vi "Begin.vi"(8 "error in (no error)":errorcluster, 11 "Dev Grabber in":refnum<class "Dev Grabber.lvclass">) -> (0 "error out":errorcluster, 3 "Dev Grabber out":refnum<class "Dev Grabber.lvclass">)   [LabVIEW 2014, in "Dev Grabber.lvlib" / "Dev Grabber.lvclass"]
uses:
  Dev Grabber.lvclass
  <vilib>/Rock Robotics/WPI/CAN/TalonSRX/WPI_CANTalonSRX_APIControlMode.ctl
  Dev Grabber.lvclass/Dev Grabber.ctl
  <vilib>/Rock Robotics/WPI/Solenoid/WPI_SolenoidOpenDouble.vi
  <vilib>/Rock Robotics/WPI/MotorControl/WPI_MotorControlOpenCANTalonSRX.vi
  Robot/Grabber/Grabber Class/Grabber.lvclass
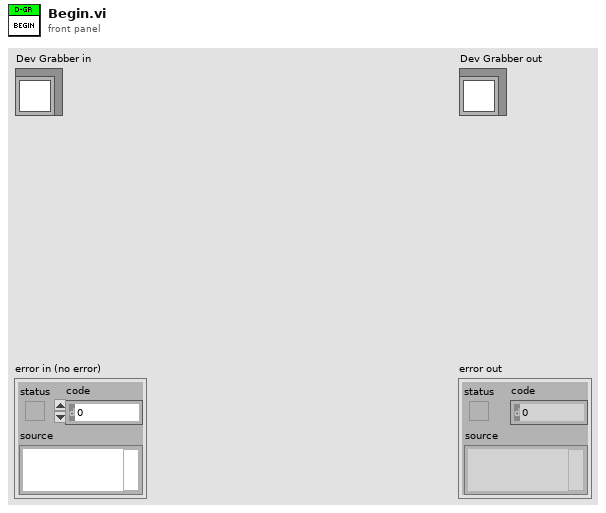
[diagram p1: front panel]
types:
  T1 = typedef "WPI_CANTalonSRX_APIControlMode.ctl" = enum8{"Percent VBus", "Speed", "Position", "Slave", "Unchanged / Invalid"}
  T2 = typedef "WPI_SolenoidChannel.ctl" = enum8{"Solenoid 0", "Solenoid 1", "Solenoid 2", "Solenoid 3", "Solenoid 4", "Solenoid 5", "Solenoid 6", "Solenoid 7", "Invalid"}
  T3 = typedef "WPI_SolenoidDevRef.ctl" = cluster{"DevStatus":errorcluster, "Pneumatics Control Module":u8, "Forward Solenoid Channel":T2, "Reverse Solenoid Channel":T2}
  T4 = typedef "WPI_MotorControlDeviceRef.ctl" = cluster{"DeviceStatus":errorcluster, "Type":T5, "PWM":cluster{"Controller":T6, "PWM Channel":T7, "DeadBand":T8}, "CAN":cluster{"Device Number":u8, "Control Mode":T9, "Semaphore":T10, "Max Vout":dbl, "TalonSRX Control Mode":T1}, "Invert":bool, "TransformRef":T11, "InvTransformRef":T11}
  T5 = typedef "WPI_MotorControlType.ctl" = enum16{"PWM", "CAN", "CANTalonSRX"}
  T6 = typedef "FPGA_TypedefDigitalModule.ctl" = enum16{"Controller 1"}
  T7 = typedef "FPGA_DIOPWMChannel.ctl" = enum8{"PWM 0", "PWM 1", "PWM 2", "PWM 3", "PWM 4", "PWM 5", "PWM 6", "PWM 7", "PWM 8", "PWM 9", "PWM MXP 0", "PWM MXP 1", "PWM MXP 2", "PWM MXP 3", "PWM MXP 4", "PWM MXP 5", "PWM MXP 6", "PWM MXP 7", "PWM MXP 8", "PWM MXP 9", "Invalid"}
  T8 = typedef "WPI_PWMDeadband.ctl" = cluster{"Name":string, "maxPositivePwm":i32, "minPositivePwm":i32, "centerPwm":i32, "maxNegativePwm":i32, "minNegativePwm":i32, "angularRange":u16}
  T9 = typedef "WPI_CANJaguar_ControlMode.ctl" = enum8{"Percent VBus", "Current", "Speed", "Position", "Voltage"}
  T10 = typedef "Semaphore RefNum" = refnum<k1>
  T11 = typedef "WPI_PWMTransform_ConPane.ctl" = refnum<vi>
  T12 = typedef "Dev Grabber.lvlib/Dev Grabber.lvclass/Dev Grabber Config.ctl" = cluster{"PCM CAN ID":u8, "Forward Solenoid Channel":T2, "Reverse Solenoid Channel":T2, "Left Motor CAN ID":u8, "Right Motor CAN ID":u8, "Left Motor Invert":bool, "Right Motor Invert":bool}
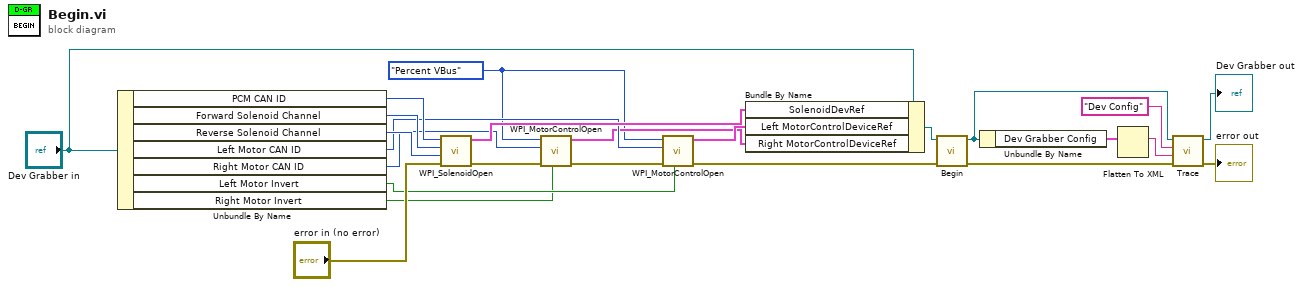
[diagram p0: block diagram]
diagram:
  w11 = WPI_CANTalonSRX_APIControlMode."Percent VBus" ("Control Mode")
  n1 = Unbundle By Name("Dev Grabber in") -> ("PCM CAN ID"=w23:u8, "Forward Solenoid Channel"=w22:T2, "Reverse Solenoid Channel"=w21:T2, "Left Motor CAN ID"=w17:u8, "Right Motor CAN ID"=w14:u8, "Left Motor Invert"=w16:bool, "Right Motor Invert"=w13:bool)
  n2 = call-poly <vilib>:"WPI_SolenoidOpen.vi"("error in (no error)"="error in (no error)", "Reverse Solenoid Channel"=w21, "Forward Solenoid Channel"=w22, "Pneumatics Control Module (0)"=w23) -> ("error out"=w10:errorcluster, "SolenoidDevRef"=w19:T3)  [unwired: 6 in]
  n3 = call-poly <vilib>:"WPI_MotorControlOpen.vi"("Invert"=w13, "error in (no error)"=w10, "Device Number"=w14, "Control Mode"=w11) -> ("error out"=w9:errorcluster, "MotorControlDeviceRef"=w12:T4)  [unwired: 6 in]
  n4 = call-poly <vilib>:"WPI_MotorControlOpen.vi"("Invert"=w16, "error in (no error)"=w9, "Device Number"=w17, "Control Mode"=w11) -> ("error out"=w8:errorcluster, "MotorControlDeviceRef"=w15:T4)  [unwired: 6 in]
  n5 = Bundle By Name(cluster="Dev Grabber in", "SolenoidDevRef"=w19, "Left MotorControlDeviceRef"=w15, "Right MotorControlDeviceRef"=w12) -> (w20:refnum<class "Dev Grabber.lvclass">)
  n6 = call-parent "Begin.vi"("error in (no error)"=w8, "System Actor in"=w20) -> ("error out"=w6:errorcluster, "System Actor out"=w3:refnum<class "Dev Grabber.lvclass">)  [unwired: 8 in]
  n7 = Unbundle By Name(w3) -> ("Dev Grabber Config"=w2:T12)
  n8 = Flatten To XML(anything=w2) -> (xml string=w1:string)
  n9 = call-dynamic "Trace.vi"("error in (no error)"=w6, "System Message"=w1, "System Action"="Dev Config", "System Actor in"=w3) -> ("error out"=→"error out":errorcluster, "System Actor out"=→"Dev Grabber out":refnum<class "Dev Grabber.lvclass">)  [unwired: 6 in]
